vi "Scale - molecular.vi"() -> ()   [LabVIEW 2016, in "features.lvlib"]
doc: "This VI takes the current values from the beamline magnetic elements and scales from the current isotope to another isotope. For atomic injection, only the masses of the isotopes are required. For molecular injection, the molecular masses, terminal voltage, stripped charge state, and pre-acc voltage are required as well."
uses:
  Features/features/features.lvlib
  controls/scale states.ctl
  <vilib>/Utility/miscctls.llb/LVRowAndColumnTypeDef.ctl
  Beam Line Sections/R45.vi
  Transmission/transmission.lvlib
  R30/R30  library.lvlib
  sub-VIs/sub-VIs.lvlib
  High energy end/High energy llb.lvlib
  controls/beamline sections.lvlib
panel:
  out "Extractor Voltage":dbl
  out "Molecular scale calc error":errorcluster
  out "Velocity scaling factor":dbl
  out "Momentum scaling factor":dbl
  in  "Terminal Voltage":dbl=8.0
  out "Pre-Acc Voltage":dbl
  in  "Low End Acc":enum32{"Setpoint", "Readback"}(radio)
  in  "Charge State":u8=3
  in  "Current/Desired Masses":i32(listbox)
  out "Scaling History":string[][](table)=[["10", "26"], ["9", "25"]]
  in  "Injection type":enum32{"Atomic", "Molecular"}(radio)=enum."Molecular"
  out "Mol Scaling Table":i32(listbox)
  out "Get values error":errorcluster
  in  "Un-scale":bool
  in  "Scale all":bool
  in  "stop":bool
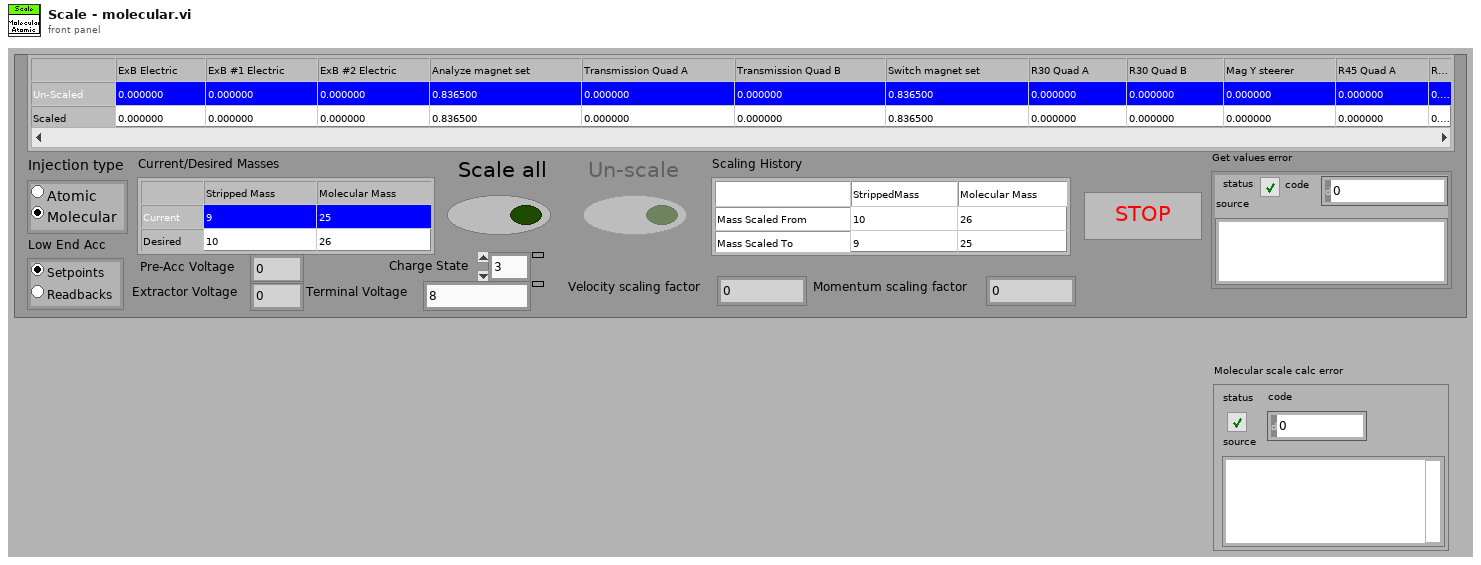
[diagram p1: front panel]
types:
  T1 = typedef "scale states.ctl" = enum16{"wait", "scale", "reset mass bkgd"}
  T2 = enum8{"Enabled", "Disabled", "Disabled and Grayed Out"}
  T3 = typedef "LVRowAndColumnTypeDef.ctl" = cluster{"Row":i32, "Column":i32}
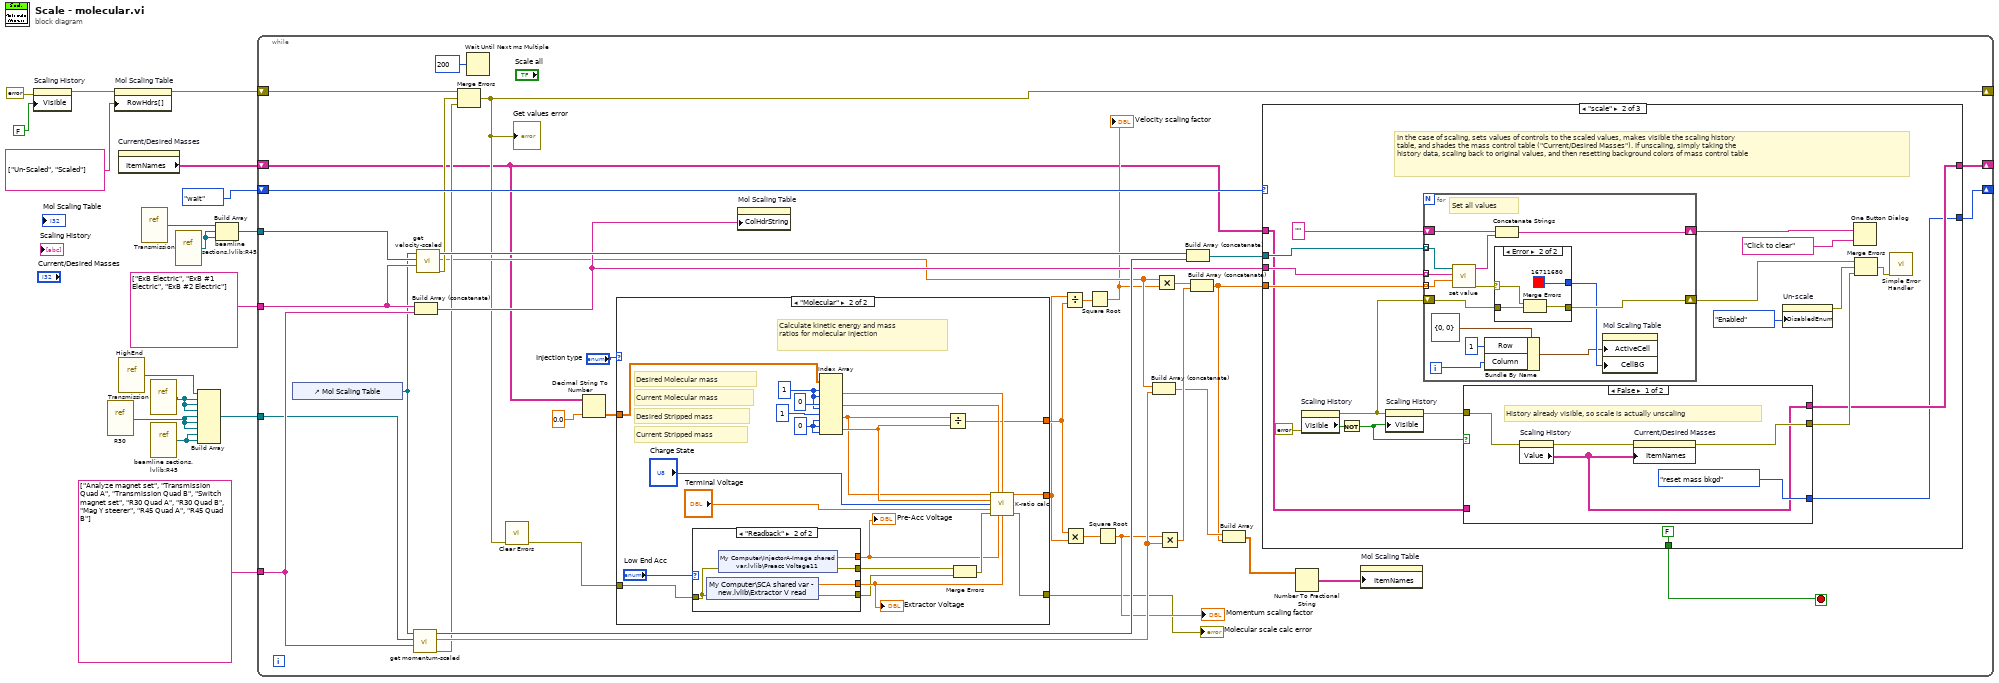
[diagram p0: block diagram]
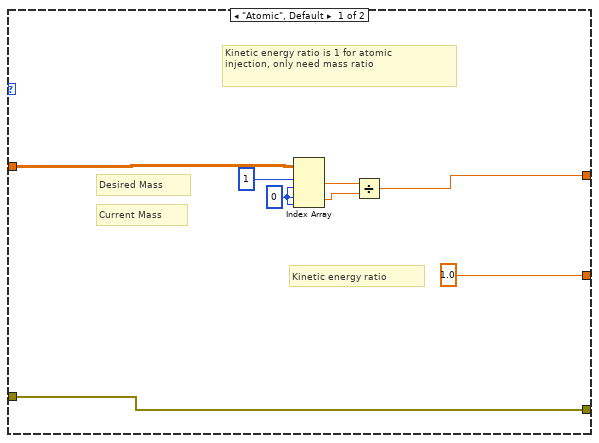
[diagram p2: hidden frame]
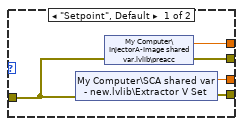
[diagram p3: hidden frame]
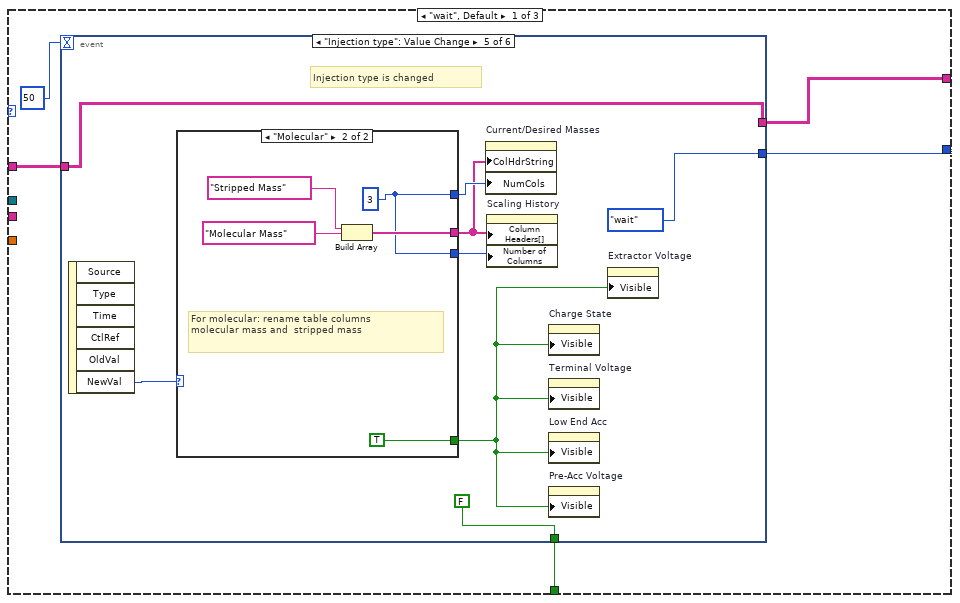
[diagram p4: hidden frame]
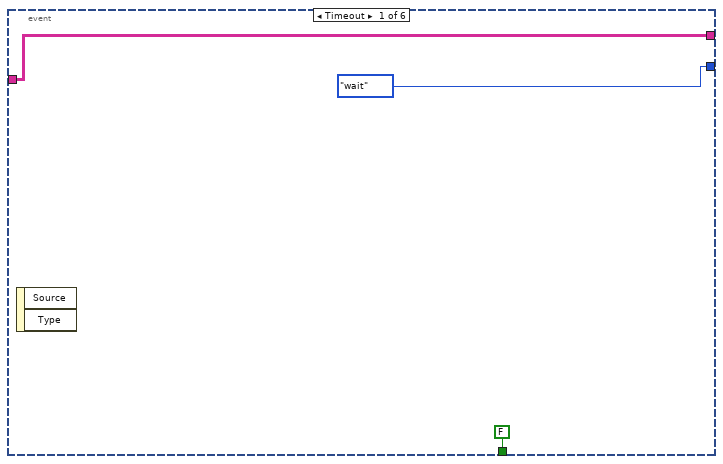
[diagram p5: hidden frame]
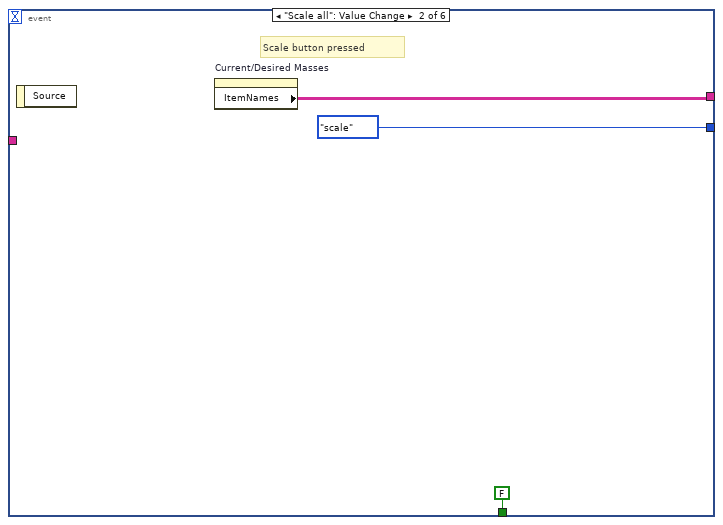
[diagram p6: hidden frame]
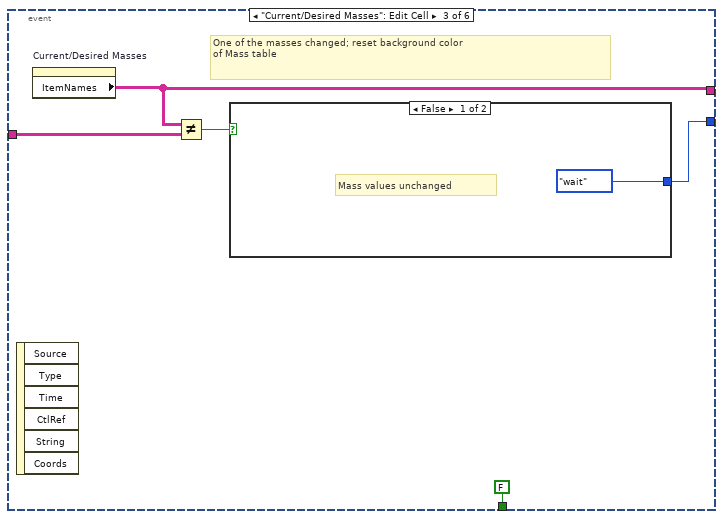
[diagram p7: hidden frame]
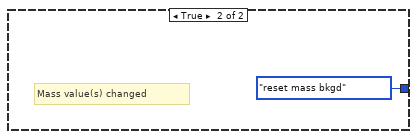
[diagram p8: hidden frame]
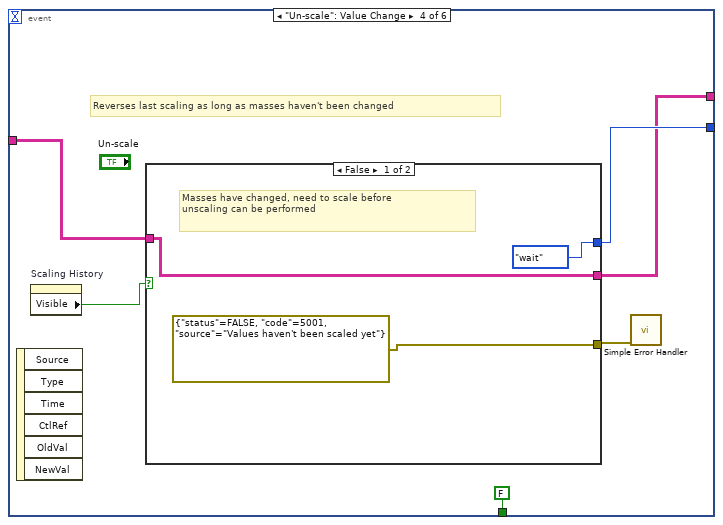
[diagram p9: hidden frame]
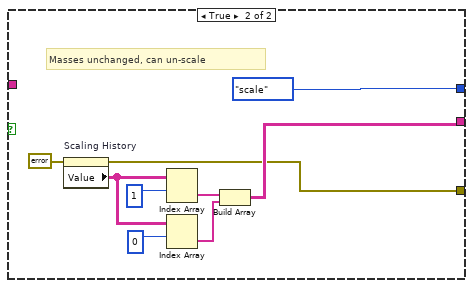
[diagram p10: hidden frame]
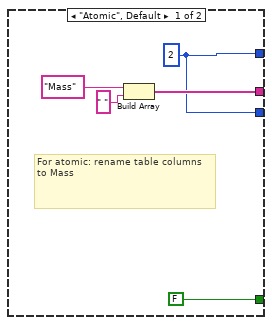
[diagram p11: hidden frame]
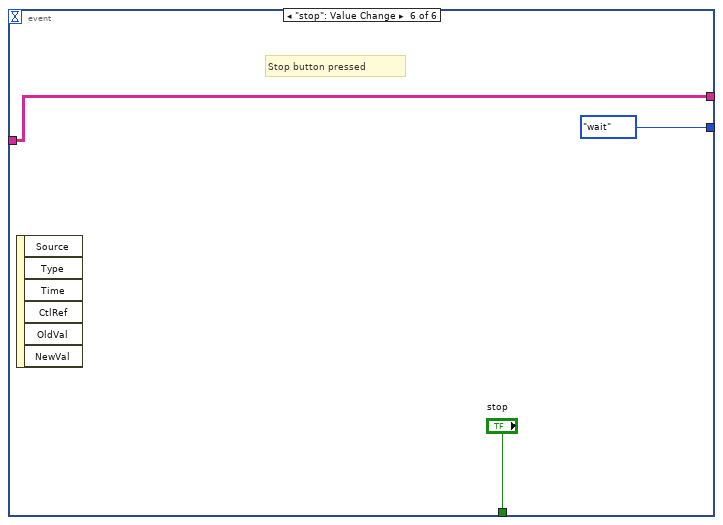
[diagram p12: hidden frame]
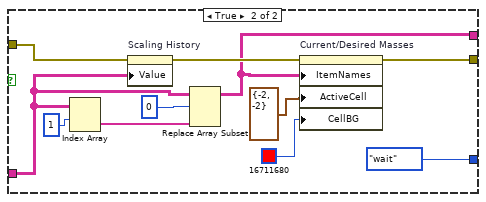
[diagram p13: hidden frame]
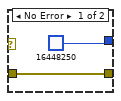
[diagram p14: hidden frame]
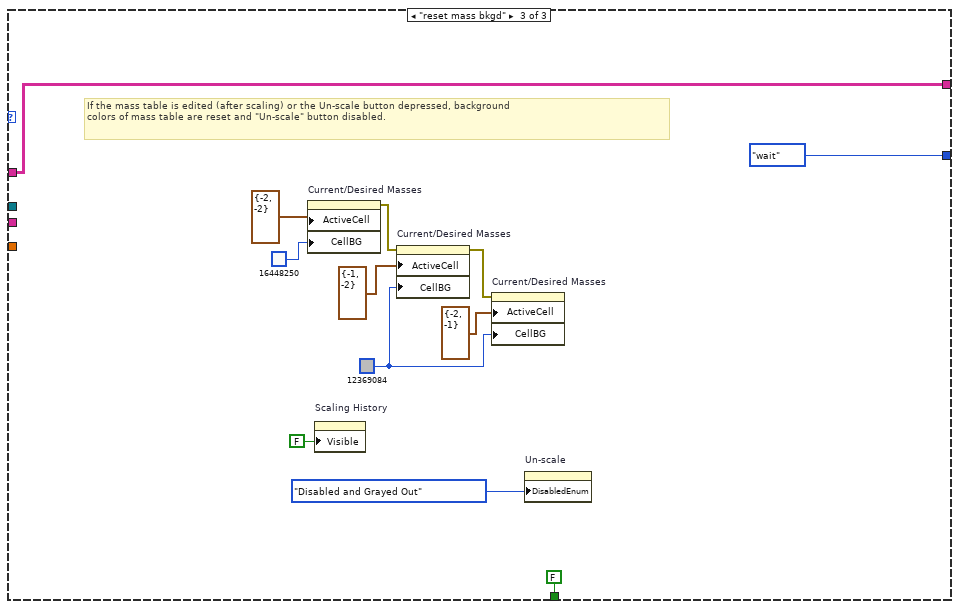
[diagram p15: hidden frame]
diagram:
  n1 = property on="Scaling History" class="Tbl (strict)"(error in=errorcluster {"status"=FALSE, "code"=0, "source"=""} ("error out"), "Visible"=FALSE) -> (error out=w2:errorcluster)  [unwired: 1 in, 1 out]
  n2 = vi-ref "R30.vi"() -> (w3:refnum<vi>)
  n3 = property on="Mol Scaling Table" class="MCListbox (strict)"(error in=w2, "RowHdrs[]"=string[] ["Un-Scaled", "Scaled"]) -> (error out=w9:errorcluster)  [unwired: 1 in, 1 out]
  n4 = property on="Current/Desired Masses" class="MCListbox (strict)"() -> ("ItemNames"=w1:string[][])  [unwired: 2 in, 2 out]
  n5 = vi-ref "HighEnd.vi"() -> (w11:refnum<vi>)
  n6 = vi-ref "Transmission.vi"() -> (w14:refnum<vi>)
  n7 = vi-ref "Transmission.vi"() -> (w12:refnum<vi>)
  n8 = vi-ref "beamline sections.lvlib:R45.vi"() -> (w4:refnum<vi>)
  n9 = vi-ref "beamline sections.lvlib:R45.vi"() -> (w15:refnum<vi>)
  n10 = Build Array(w11, w12, w12, w12, w3, w3, w3, w4, w4) -> (w10:refnum<vi>[])
  n11 = Build Array(w14, w15, w15) -> (w13:refnum<vi>[])
  n12 = while {
    shift-right: [w24] -> _
    shift-left: w9 -> [w48]
    tunnel: string[] ["Analyze magnet set", "Transmission Quad A", "Transmission Quad B", "Switch magnet set", "R30 Quad A", "R30 Quad B", "Mag Y steerer", "R45 Quad A", "R45 Quad B"] -> [w47]
    tunnel: string[] ["ExB Electric", "ExB #1 Electric", "ExB #2 Electric"] -> [w39]
    tunnel: w13 -> [w46]
    tunnel: w10 -> [w36]
    shift-right: [w25] -> _
    shift-left: scale_states."wait" -> [w42]
    shift-right: [w19] -> _
    shift-left: w1 -> [w18]
    stop <- w20 stop-if-true
    n13 = control-ref of="Mol Scaling Table"() -> (w21:refnum<vi>)
    n14 = call "get momentum-scaled.vi"("Array 2"=w47, "Array"=w36, "MulticolumnListbox in"=w21) -> ("error out"=w41:errorcluster, "Array 3"=w51:ext[], "Array 4"=w52:refnum<vi>[])  [unwired: 6 in]
    n15 = Build Array (concatenate)(w39, w47) -> (w49:string[])
    n16 = call "get velocity-scaled.vi"("Array"=w39, "Array 2"=w46, "MulticolumnListbox in"=w21) -> ("error out"=w40:errorcluster, "Array 3"=w32:ext[], "Array 4"=w53:refnum<vi>[])  [unwired: 6 in]
    n17 = Merge Errors(w48, w40, w41) -> (w24:errorcluster)
    "Get values error" <- w24
    n18 = Wait Until Next ms Multiple(millisecond multiple=u32 200) -> ()  [unwired: 1 out]
    n19 = call <vilib>:"Clear Errors.vi"("error in (no error)"=w24) -> ("error out"=w23:errorcluster)  [unwired: 5 in, 1 out]
    n20 = Decimal String To Number(string=w18, default (0L)=0.0 ("default (0 I32)")) -> (number=w35:dbl[][])  [unwired: 1 in, 1 out]
    n21 = case shown="\"Molecular\"" "Injection type" {
      tunnel: w35 -> [w59 w82]
      tunnel: [w57 w75] -> w29
      tunnel: [1.0 w74] -> w28
      tunnel: w23 -> [w56 w72]
      tunnel: [w56 w73] -> w22
      frame "Atomic", Default {
        w62 = 0 ("index (row)")
        # "Kinetic energy ratio is 1 for atomic\ninjection, only need mass ratio"
        # "Kinetic energy ratio"
        # "Desired Mass"
        # "Current Mass"
        n22 = Index Array(array=w59, index (row) #1=1 ("index (row)"), index (col) #1=w62, index (row) #2=w62, index (col) #2=w62) -> (element #1=w61:dbl, element #2=w60:dbl)
        n23 = Divide(x=w61, y=w60) -> (x/y=w57:dbl)
      }
      frame "Molecular" {
        w70 = 0 ("index (row)")
        w71 = 1 ("index (row)")
        # "Calculate kinetic energy and mass\nratios for molecular injection"
        # "Desired Stripped mass"
        # "Desired Molecular mass"
        # "Current Stripped mass"
        # "Current Molecular mass"
        n24 = case shown="\"Readback\"" "Low End Acc" {
          tunnel: [w89 w94] -> w67
          tunnel: w72 -> [w87 w90]
          tunnel: [w88 w93] -> w65
          tunnel: [w85 w92] -> w66
          tunnel: [w86 w91] -> w64
          frame "Setpoint", Default {
            n25 = shared-variable "My Computer\\SCA shared var - new.lvlib\\Extractor V Set"(error in=w87) -> (w85:dbl, error out=w86:errorcluster)
            n26 = shared-variable "My Computer\\InjectorA-Image shared var.lvlib\\preacc"(error in=w87) -> (w89:dbl, error out=w88:errorcluster)
          }
          frame "Readback" {
            n27 = shared-variable "My Computer\\SCA shared var - new.lvlib\\Extractor V read"(error in=w90) -> (w92:dbl, error out=w91:errorcluster)
            n28 = shared-variable "My Computer\\InjectorA-Image shared var.lvlib\\Preacc Voltage11"(error in=w90) -> (w94:dbl, error out=w93:errorcluster)
          }
        }
        "Pre-Acc Voltage" <- w67
        "Extractor Voltage" <- w66
        n29 = Index Array(array=w82, index (row) #1=w71, index (col) #1=w71, index (row) #2=0 ("index (row)"), index (col) #2=w71, index (row) #3=1 ("index (row)"), index (col) #3=w70, index (row) #4=w70, index (col) #4=w70) -> (element #1=w76:dbl, element #2=w77:dbl, element #3=w78:dbl, element #4=w79:dbl)
        n30 = Divide(x=w78, y=w79) -> (x/y=w75:dbl)
        n31 = Merge Errors(w65, w64) -> (w69:errorcluster)
        n32 = call "K-ratio calc.vi"("Desired Stripped mass"=w78, "Current Molecular Mass"=w77, "Desired Molecular Mass"=w76, "Current Stripped Mass"=w79, "Charge State"="Charge State", "Terminal Voltage"="Terminal Voltage", "error in"=w69, "PreAcc Voltage"=w67, "Extractor Voltage"=w66) -> ("Kinetic energy ratio"=w74:dbl, "error out"=w73:errorcluster)  [unwired: 5 in]
      }
    }
    "Molecular scale calc error" <- w22
    n33 = property on="Mol Scaling Table" class="MCListbox (strict)"("ColHdrString"=w49) -> ()  [unwired: 2 in, 2 out]
    n34 = Divide(x=w28, y=w29) -> (x/y=w31:dbl)
    n35 = Multiply(x=w29, y=w28) -> (x*y=w30:dbl)
    n36 = Square Root(x=w31) -> (sqrt(x)=w27:dbl)
    "Velocity scaling factor" <- w27
    n37 = Square Root(x=w30) -> (sqrt(x)=w26:dbl)
    "Momentum scaling factor" <- w26
    n38 = Build Array (concatenate)(w32, w51) -> (w45:ext[])
    n39 = Multiply(x=w32, y=w27) -> (x*y=w55:ext[])
    n40 = Multiply(x=w26, y=w51) -> (x*y=w54:ext[])
    n41 = Build Array (concatenate)(w53, w52) -> (w50:refnum<vi>[])
    n42 = Build Array (concatenate)(w55, w54) -> (w44:ext[])
    n43 = Build Array(w45, w44) -> (w37:ext[][])
    n44 = case shown="\"scale\"" w42 {
      tunnel: w50 -> [_ w168 _]
      tunnel: w49 -> [_ w167 _]
      tunnel: w44 -> [_ w166 _]
      tunnel: [w98 w152 scale_states."wait"] -> w25
      tunnel: [w97 FALSE ("stop") FALSE ("stop")] -> w20
      tunnel: w18 -> [w96 w159 w208]
      tunnel: [w95 w155 w208] -> w19
      frame "wait", Default {
        n45 = event shown="[4] \"Injection type\": Value Change" {
          selector: _ -> [_ _ _ _ _ _]
          dyn-events: _ -> [_ _ _ _ _ _]
          timeout: 50 -> [_ _ _ _ _ _]
          tunnel: [scale_states."wait" scale_states."scale" w106 w118 scale_states."wait" scale_states."wait"] -> w98
          tunnel: [FALSE ("stop") FALSE ("stop") FALSE ("stop") FALSE ("stop") FALSE ("stop") "stop"] -> w97
          tunnel: w96 -> [w100 _ w108 w114 w132 w149]
          tunnel: [w100 w103 w107 w113 w132 w149] -> w95
          event Timeout {
            n46 = event-data() -> ()  [unwired: 1 in, 2 out]
          }
          event "Scale all": Value Change {
            # "Scale button pressed"
            n47 = event-data() -> ()  [unwired: 1 in, 1 out]
            n48 = property on="Current/Desired Masses" class="MCListbox (strict)"() -> ("ItemNames"=w103:string[][])  [unwired: 2 in, 2 out]
          }
          event "Current/Desired Masses": Edit Cell {
            # "One of the masses changed; reset background color\nof Mass table"
            n49 = event-data() -> ()  [unwired: 1 in, 6 out]
            n50 = property on="Current/Desired Masses" class="MCListbox (strict)"() -> ("ItemNames"=w107:string[][])  [unwired: 2 in, 2 out]
            n51 = Not Equal?(x=w107, y=w108) -> (x != y?=w109:bool)
            n52 = case shown="False" w109 {
              tunnel: [scale_states."wait" scale_states."reset mass bkgd"] -> w106
              frame False {
                # "Mass values unchanged"
              }
              frame True {
                # "Mass value(s) changed"
              }
            }
          }
          event "Un-scale": Value Change {
            # "Reverses last scaling as long as masses haven't been changed"
            n53 = event-data() -> ()  [unwired: 1 in, 6 out]
            n54 = property on="Scaling History" class="Tbl (strict)"() -> ("Visible"=w115:bool)  [unwired: 2 in, 2 out]
            n55 = case shown="False" w115 {
              tunnel: [scale_states."wait" scale_states."scale"] -> w118
              tunnel: [errorcluster {"status"=FALSE, "code"=5001, "source"="Values haven't been scaled yet"} ("error out") w122] -> w117
              tunnel: w114 -> [w119 _]
              tunnel: [w119 w124] -> w113
              frame False {
                # "Masses have changed, need to scale before \nunscaling can be performed"
              }
              frame True {
                # "Masses unchanged, can un-scale"
                n56 = property on="Scaling History" class="Tbl (strict)"(error in=errorcluster {"status"=FALSE, "code"=0, "source"=""} ("error out")) -> (error out=w122:errorcluster, "Value"=w123:string[][])  [unwired: 1 in, 1 out]
                n57 = Index Array(array=w123, index (row)=1) -> (element=w128:string[])  [unwired: 1 in]
                n58 = Index Array(array=w123, index (row)=0) -> (element=w129:string[])  [unwired: 1 in]
                n59 = Build Array(w128, w129) -> (w124:string[][])
              }
            }
            n60 = call <vilib>:"Simple Error Handler.vi"("error in (no error)"=w117) -> ()  [unwired: 4 in, 5 out]
          }
          event "Injection type": Value Change {
            # "Injection type is changed"
            n61 = event-data() -> ("NewVal"=w138:enum32{"Atomic", "Molecular"})  [unwired: 1 in, 5 out]
            n62 = case shown="\"Molecular\"" w138 {
              tunnel: [w141 w148] -> w134
              tunnel: [FALSE TRUE] -> w131
              tunnel: [w139 w146] -> w135
              tunnel: [w139 w146] -> w136
              frame "Atomic", Default {
                w139 = 2
                # "For atomic: rename table columns to Mass"
                n63 = Build Array("Mass", " ") -> (w141:string[])
              }
              frame "Molecular" {
                w146 = 3
                # "For molecular: rename table columns \nmolecular mass and  stripped mass"
                n64 = Build Array("Stripped Mass", "Molecular Mass") -> (w148:string[])
              }
            }
            n65 = property on="Current/Desired Masses" class="MCListbox (strict)"("ColHdrString"=w134, "NumCols"=w135) -> ()  [unwired: 2 in, 2 out]
            n66 = property on="Scaling History" class="Tbl (strict)"("Column Headers[]"=w134, "Number of Columns"=w136) -> ()  [unwired: 2 in, 2 out]
            n67 = property on="Charge State" class="DigNum (strict)"("Visible"=w131) -> ()  [unwired: 2 in, 2 out]
            n68 = property on="Terminal Voltage" class="DigNum (strict)"("Visible"=w131) -> ()  [unwired: 2 in, 2 out]
            n69 = property on="Low End Acc" class="RadioBtnsControl (strict)"("Visible"=w131) -> ()  [unwired: 2 in, 2 out]
            n70 = property on="Pre-Acc Voltage" class="DigNum (strict)"("Visible"=w131) -> ()  [unwired: 2 in, 2 out]
            n71 = property on="Extractor Voltage" class="DigNum (strict)"("Visible"=w131) -> ()  [unwired: 2 in, 2 out]
          }
          event "stop": Value Change {
            # "Stop button pressed"
            n72 = event-data() -> ()  [unwired: 1 in, 6 out]
          }
        }
      }
      frame "scale" {
        # "In the case of scaling, sets values of controls to the scaled values, makes visible the scaling history\ntable, and shades the mass control table (\"Current/Desired Masses\"). If unscaling, simply taking the \nhistory data, scaling back to original values, and then resetting background colors of mass control table"
        n73 = property on="Scaling History" class="Tbl (strict)"(error in=errorcluster {"status"=FALSE, "code"=0, "source"=""} ("error out")) -> (error out=w158:errorcluster, "Visible"=w156:bool)  [unwired: 1 in, 1 out]
        n74 = Not(x=w156) -> (.not. x?=w154:bool)
        n75 = property on="Scaling History" class="Tbl (strict)"(error in=w158, "Visible"=w154) -> (error out=w153:errorcluster)  [unwired: 1 in, 1 out]
        n76 = for {
          tunnel: w166 -> [w200] mode=indexing
          tunnel: w168 -> [w201] mode=indexing
          tunnel: w167 -> [w199] mode=indexing
          shift-right: [w196] -> w170
          shift-left: w158 -> [w197]
          shift-right: [w193] -> w164
          shift-left: "" -> [w195]
          i -> [w189]
          # "Set all values"
          n77 = call "set value.vi"("Set value"=w200, "Control Name"=w199, "VI Refnum"=w201) -> ("error out"=w198:errorcluster, "Output string"=w194:string)  [unwired: 7 in]
          n78 = Bundle By Name(cluster=T3 {"Row"=0, "Column"=0} ("Active Cell:Active Cell"), "Row"=1, "Column"=w189) -> (w190:T3)
          n79 = case shown="Error" w198 {
            selector: w198 -> [_ w205]
            tunnel: w197 -> [w203 w206]
            tunnel: [w203 w207] -> w196
            tunnel: [u32 16448250 u32 16711680] -> w192
            frame No Error {
            }
            frame Error {
              n80 = Merge Errors(w205, w206) -> (w207:errorcluster)
            }
          }
          n81 = Concatenate Strings(w195, w194) -> (w193:string)
          n82 = property on="Mol Scaling Table" class="MCListbox (strict)"("ActiveCell"=w190, "CellBG"=w192) -> ()  [unwired: 2 in, 2 out]
        }
        n83 = case shown="False" w154 {
          tunnel: [w174 w183] -> w161
          tunnel: w159 -> [_ w181]
          tunnel: w153 -> [w173 w177]
          tunnel: [w172 w179] -> w155
          tunnel: [scale_states."reset mass bkgd" ("t") scale_states."wait"] -> w152
          frame False {
            # "History already visible, so scale is actually unscaling"
            n84 = property on="Scaling History" class="Tbl (strict)"(error in=w173) -> (error out=w175:errorcluster, "Value"=w172:string[][])  [unwired: 1 in, 1 out]
            n85 = property on="Current/Desired Masses" class="MCListbox (strict)"(error in=w175, "ItemNames"=w172) -> (error out=w174:errorcluster)  [unwired: 1 in, 1 out]
          }
          frame True {
            n86 = Index Array(array=w181, index (row)=1) -> (element=w182:string[])  [unwired: 1 in]
            n87 = property on="Scaling History" class="Tbl (strict)"(error in=w177, "Value"=w181) -> (error out=w187:errorcluster)  [unwired: 1 in, 1 out]
            n88 = Replace Array Subset(array=w181, new element=w182, index (row)=0) -> (w179:string[][])  [unwired: 1 in]
            n89 = property on="Current/Desired Masses" class="MCListbox (strict)"(error in=w187, "ItemNames"=w179, "ActiveCell"=T3 {"Row"=-2, "Column"=-2} ("Active Cell:Active Cell"), "CellBG"=u32 16711680) -> (error out=w183:errorcluster)  [unwired: 1 in, 1 out]
          }
        }
        n90 = property on="Un-scale" class="Bool"("DisabledEnum"=T2."Enabled" ("Disabled")) -> (error out=w169:errorcluster)  [unwired: 2 in, 1 out]
        n91 = One Button Dialog(message=w164, button name ("OK")="Click to clear") -> ()  [unwired: 1 out]
        n92 = Merge Errors(w170, w169, w161) -> (w162:errorcluster)
        n93 = call <vilib>:"Simple Error Handler.vi"("error in (no error)"=w162) -> ()  [unwired: 4 in, 5 out]
      }
      frame "reset mass bkgd" {
        w211 = u32 12369084 ("Active Cell:Cell Background Color")
        # "If the mass table is edited (after scaling) or the Un-scale button depressed, background \ncolors of mass table are reset and \"Un-scale\" button disabled."
        n94 = property on="Current/Desired Masses" class="MCListbox (strict)"("ActiveCell"=T3 {"Row"=-2, "Column"=-2} ("Active Cell:Active Cell"), "CellBG"=u32 16448250) -> (error out=w213:errorcluster)  [unwired: 2 in, 1 out]
        n95 = property on="Scaling History" class="Tbl (strict)"("Visible"=FALSE) -> ()  [unwired: 2 in, 2 out]
        n96 = property on="Current/Desired Masses" class="MCListbox (strict)"(error in=w213, "ActiveCell"=T3 {"Row"=-1, "Column"=-2} ("Active Cell:Active Cell"), "CellBG"=w211) -> (error out=w214:errorcluster)  [unwired: 1 in, 1 out]
        n97 = property on="Current/Desired Masses" class="MCListbox (strict)"(error in=w214, "ActiveCell"=T3 {"Row"=-2, "Column"=-1} ("Active Cell:Active Cell"), "CellBG"=w211) -> ()  [unwired: 1 in, 2 out]
        n98 = property on="Un-scale" class="Bool"("DisabledEnum"=T2."Disabled and Grayed Out" ("Disabled")) -> ()  [unwired: 2 in, 2 out]
      }
    }
    n99 = Number To Fractional String(number=w37) -> (F-format string=w38:string[][])  [unwired: 3 in]
    n100 = property on="Mol Scaling Table" class="MCListbox (strict)"("ItemNames"=w38) -> ()  [unwired: 2 in, 2 out]
  }
